vi "MakeExample.vi"(8 "error in (no error)":errorcluster, 9 "TriggerRefractoryPeriod (Frames)":i32, 10 "StimulusObject Parameters":variant, 11 "HeadTailContinuousGWN in":refnum<class "HeadTailContinuousGWN.lvclass">) -> (0 "error out":errorcluster, 3 "HeadTailContinuousGWN out":refnum<class "HeadTailContinuousGWN.lvclass">)   [LabVIEW 2019, in "HeadTailContinuousGWN.lvclass"]
uses:
  HeadTailContinuousGWN.lvclass
  HeadTailContinuousGWNInputCluster.ctl
  HeadTailContinuousGWN.lvclass/HeadTailContinuousGWN.ctl
  ParametersGlobal.vi
  StimulusObject.lvclass
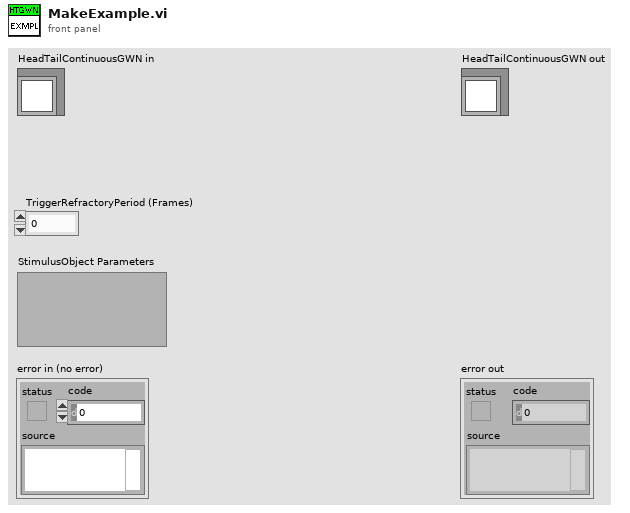
[diagram p1: front panel]
types:
  T1 = typedef "HeadTailContinuousGWN.lvclass/HeadTailContinuousGWNInputCluster.ctl" = cluster{"offset (red uW/mm^2m, blue is negative)":sgl, "correlation time (s)":sgl, "standard deviation (red uW/mm^2)":sgl, "Max blue stimulus (uW/mm^2)":sgl, "Max red stimulus (uW/mm^2)":sgl, "dot radius (mm)":sgl}
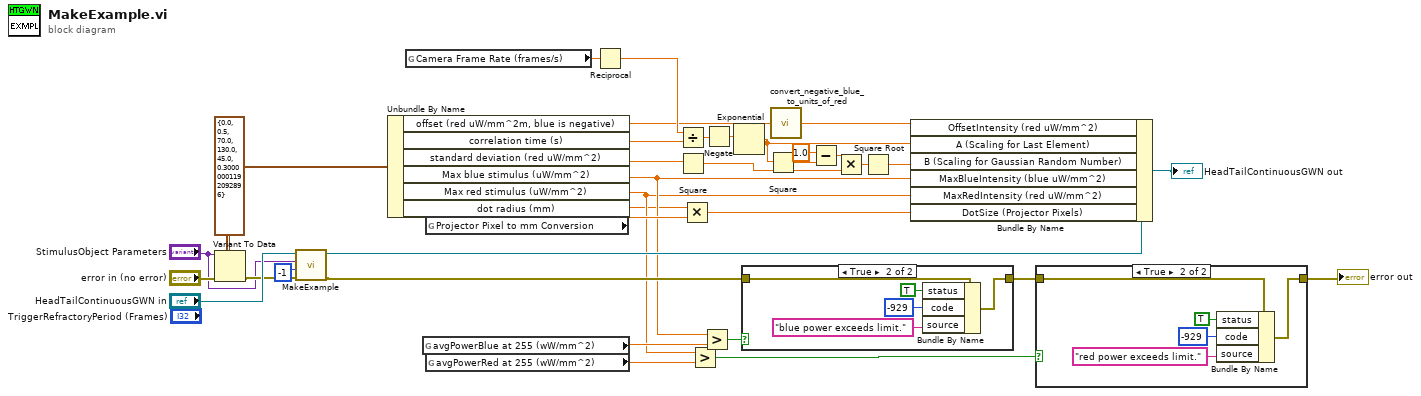
[diagram p0: block diagram]
diagram:
  n1 = Variant To Data(error in="error in (no error)", type=T1 {"offset (red uW/mm^2m, blue is negative)"=0.0, "correlation time (s)"=0.5, "standard deviation (red uW/mm^2)"=70.0, "Max blue stimulus (uW/mm^2)"=130.0, "Max red stimulus (uW/mm^2)"=45.0, "dot radius (mm)"=0.3} ("HeadTailContinousGWNInputCluser"), Variant="StimulusObject Parameters") -> (data=w12:T1, error out=w10:errorcluster)
  n2 = call-parent "MakeExample.vi"("error in (no error)"=w10, "TriggerRefractoryPeriod (Frames)"=-1, "StimulusObject Parameters"="StimulusObject Parameters", "StimulusObject in"="HeadTailContinuousGWN in") -> ("error out"=w18:errorcluster, "StimulusObject out"=w35:refnum<class "HeadTailContinuousGWN.lvclass">)  [unwired: 6 in]
  n3 = Unbundle By Name(w12) -> ("offset (red uW/mm^2m, blue is negative)"=w2:sgl, "correlation time (s)"=w9:sgl, "standard deviation (red uW/mm^2)"=w8:sgl, "Max blue stimulus (uW/mm^2)"=w7:sgl, "Max red stimulus (uW/mm^2)"=w6:sgl, "dot radius (mm)"=w5:sgl)
  n4 = global read "ParametersGlobal.vi" "Camera Frame Rate (frames/s)"() -> (w25:sgl)
  n5 = global read "ParametersGlobal.vi" "avgPowerBlue at 255 (wW/mm^2)"() -> (w20:sgl)
  n6 = global read "ParametersGlobal.vi" "Projector Pixel to mm Conversion"() -> (w24:sgl)
  n7 = global read "ParametersGlobal.vi" "avgPowerRed at 255 (wW/mm^2)"() -> (w19:sgl)
  n8 = Reciprocal(x=w25) -> (1/x=w27:sgl)
  n9 = Divide(x=w27, y=w9) -> (x/y=w28:sgl)
  n10 = Square(x=w8) -> (x^2=w32:sgl)
  n11 = Multiply(x=w5, y=w24) -> (x*y=w23:sgl)
  n12 = Greater?(x=w6, y=w19) -> (0:w14:bool)
  n13 = Greater?(x=w7, y=w20) -> (0:w17:bool)
  n14 = Negate(x=w28) -> (-x=w29:sgl)
  n15 = Exponential(1:w29) -> (0:w22:sgl)
  n16 = case shown="True" w17 {
    tunnel: w18 -> [w37 w42]
    tunnel: [w37 w41] -> w16
    frame False {
    }
    frame True {
      n17 = Bundle By Name(cluster=w42, "status"=TRUE, "code"=-929, "source"="blue power exceeds limit.") -> (w41:errorcluster)
    }
  }
  n18 = Square(x=w22) -> (x^2=w30:sgl)
  n19 = call "convert_negative_blue_to_units_of_red.vi"("Intensity in units of red (positive) and blue (negative)"=w2) -> ("Intensity in units of red (positive and negative)"=w1:sgl)
  n20 = Subtract(x=sgl 1.0, y=w30) -> (x-y=w31:sgl)
  n21 = Multiply(x=w31, y=w32) -> (x*y=w33:sgl)
  n22 = Square Root(x=w33) -> (sqrt(x)=w21:sgl)
  n23 = Bundle By Name(cluster=w35, "OffsetIntensity (red uW/mm^2)"=w1, "A (Scaling for Last Element)"=w22, "B (Scaling for Gaussian Random Number)"=w21, "MaxBlueIntensity (blue uW/mm^2)"=w7, "MaxRedIntensity (red uW/mm^2)"=w6, "DotSize (Projector Pixels)"=w23) -> (→"HeadTailContinuousGWN out":refnum<class "HeadTailContinuousGWN.lvclass">)
  n24 = case shown="True" w14 {
    tunnel: w16 -> [w43 w48]
    tunnel: [w43 w47] -> w15
    frame False {
    }
    frame True {
      n25 = Bundle By Name(cluster=w48, "status"=TRUE, "code"=-929, "source"="red power exceeds limit.") -> (w47:errorcluster)
    }
  }
  "error out" <- w15
